vi "Dispose Reference.vi"(8 "error in (no error)":errorcluster, 11 "Generic Reference":refnum<data-value>) -> (0 "error out":errorcluster)   [LabVIEW 2013, in "Hierarchy Framework.lvlib" / "Generic.lvclass"]
uses:
  Generic.lvclass
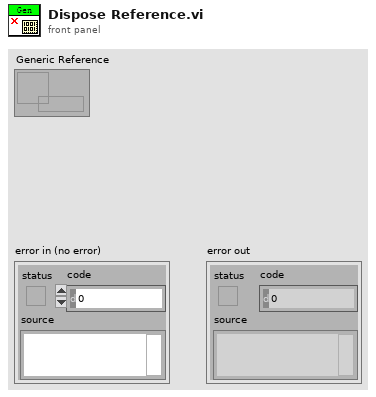
[diagram p1: front panel]
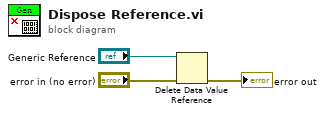
[diagram p0: block diagram]
diagram:
  n1 = Delete Data Value Reference(data value reference="Generic Reference", error in="error in (no error)") -> (error out=→"error out":errorcluster)  [unwired: 1 out]
